vi "ADAM_kernal_server.vi"(0 "Board type":T2=enum."NB-MIO-16H", 1 "interval scanning":bool, 2 "Client Time":dbl, 5 "No of samples+extra":i32=128 min=0 step=1, 7 "Trigger mode":T1, 9 "output polarity":u16(ring)=1 items=["do not change", "positive", "negative"], 11 "Ch & spans":T3[](array[typedef]) {"low limit (-10V)" format="%.3f"; "high limit (10V)" format="%.3f"}, 12 "Actual Sampling rate (Hz)":dbl=1000.0 format="%.2f", 13 "Local Client?":bool, 14 "Current Block No":i32) -> (4 "I16 data":i16[][](array[numeric]), 6 "Block Timings":T4={"Started"=0.0, "Ended"=0.0, "Analogue Frequency Hz"=1000.0} {"Analogue Frequency Hz" format="%.2f"}, 10 "group channel settings":T5(array[cluster]) {"scale offset" format="%.2f"; "scale multiplier" format="%.2f"; "gain" format="%.2f"; "range" format="%.2f"; "lower input limits" format="%.2f"; "upper input limits" format="%.2f"}, 15 "error out":errorcluster)   [LabVIEW 2010]
uses:
  ADAM_Global.vi
  Anemometry/Anemometry Sub Vis/Globals/Meas_global.vi
  Anemometry/Anemometry Sub Vis/Controls/Block_start_and_end.ctl
  Channel_Description_Global.vi
  Anemometry/Anemometry Sub Vis/Globals/Constants_global.vi
  Anemometry/Anemometry Sub Vis/Controls/Board_Types.ctl
  Anemometry/Anemometry Sub Vis/Controls/Ch_and_Spans.ctl
  Anemometry/Anemometry Sub Vis/Controls/Trigger_Mode.ctl
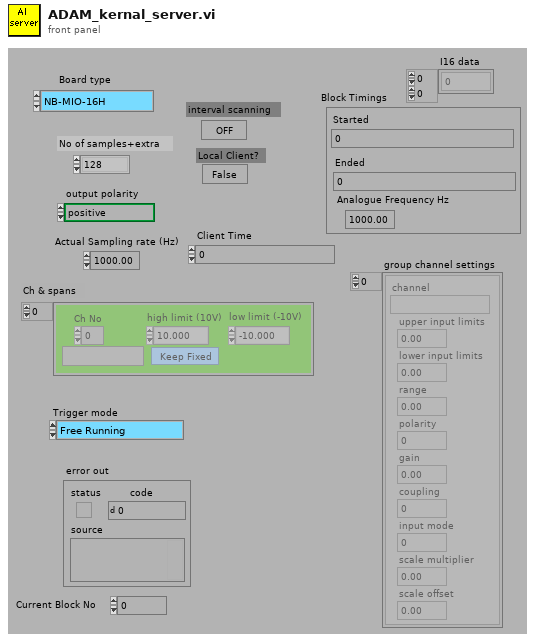
[diagram p1: front panel]
types:
  T1 = typedef "Trigger_Mode.ctl" = enum16{"Free Running", "Start on Trigger", "Trigger Every Block", "Trigger Every Sample"}
  T2 = typedef "Board_Types.ctl" = enum16{"Simulate", "NB-MIO-16H", "PCI-MIO-16E", "6000E Series", "USB-92xx", "ADC488", "Lab-NB", "NB-DIO-24", "NI-DAQmx", "Local ADAM", "Server Channels"}
  T3 = typedef "Ch_and_Spans.ctl" = cluster{"high limit (10V)":sgl, "low limit (-10V)":sgl, "Ch No":i16, "Var name":string, "Use Latest Calib":bool}
  T4 = typedef "Block_start_and_end.ctl" = cluster{"Started":dbl, "Ended":dbl, "Analogue Frequency Hz":dbl}
  T5 = cluster{"channel":string, "upper input limits":sgl, "lower input limits":sgl, "range":sgl, "polarity":u16, "gain":sgl, "coupling":u16, "input mode":u16, "scale multiplier":dbl, "scale offset":dbl}[]
  T6 = cluster{"channel":string, "upper input limits":sgl, "lower input limits":sgl, "range":sgl, "polarity":u16, "gain":sgl, "coupling":u16, "input mode":u16, "scale multiplier":dbl, "scale offset":dbl}
  T7 = typedef "Ch_description_ADAM.ctl" = cluster{"Ch Name":string, "Type":T8, "Function":T9, "Ch State":T10, "Calibration type":T11, "A":dbl, "B":dbl, "C":dbl, "D":dbl, "Comments":string, "Address":T12, "String":string, "Duty":u16}
  T8 = typedef "Module_type_ADAM.ctl" = enum16{"4011", "4012", "4013", "4014", "4016", "4017", "4018", "4021", "4050", "4052", "4053", "4060", "4080", "5000", "5017", "5018", "5024", "5051", "5056", "5060", "6060", "Tracker", "WEST", "GILL", "JEM", "VICI", "Vaisala", "DRUCK", "Run VI Named:", "IR2100", "PPT", "Comparator", "VIRTUAL", "Hold Value", "Read A", "Read Ch", "Coded", "Client Info", "Web Client", "X10", "Test"}
  T9 = typedef "Function_ADAM.ctl" = enum16{"Analogue Input", "Digital Input", "Event counter", "Event rate", "Analogue Output", "Digital Output", "Relay Output"}
  T10 = typedef "Channel_State.ctl" = enum16{"On", "Off", "Always On", "Always Off"}
  T11 = typedef "Calib_type_ADAM.ctl" = enum16{"Raw", "Bx + A", "Cx^2 + Bx + A", "Dx^3 + Cx^2 + Bx + A", "In Band", "Hi-Tec Q", "Hi-Tec M_dot", "Text"}
  T12 = typedef "Address.ctl" = cluster{"Main":i32, "Ch.":i32, "Sub":i32, "Port Name":string}
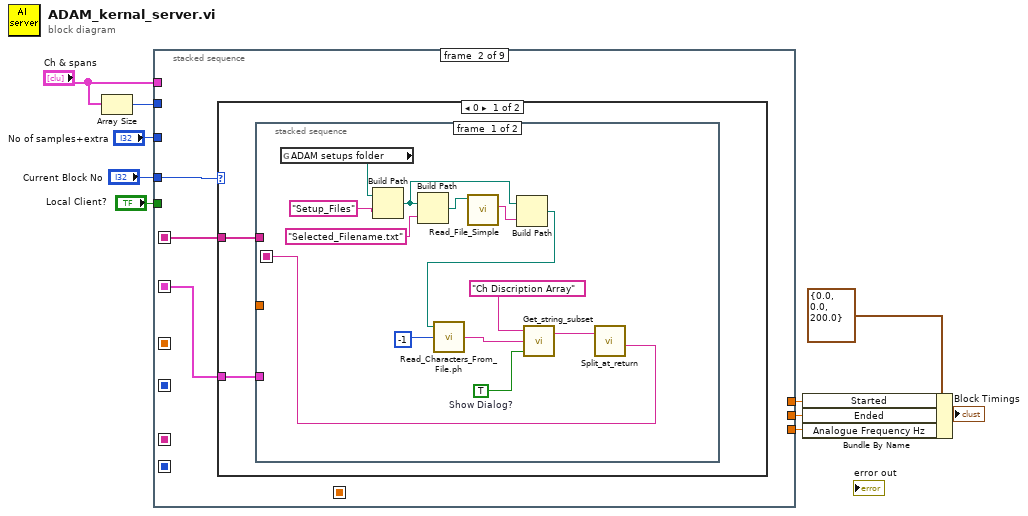
[diagram p0: block diagram]
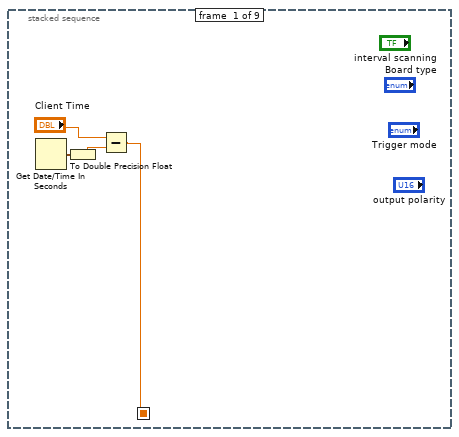
[diagram p2: hidden frame]
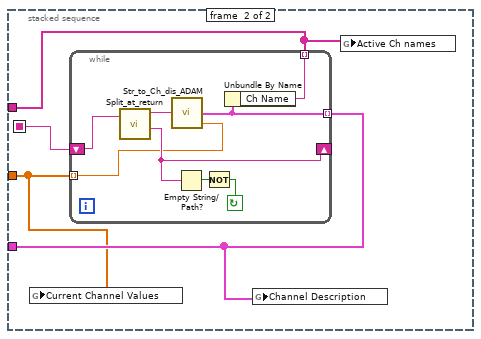
[diagram p3: hidden frame]
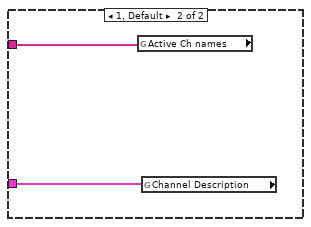
[diagram p4: hidden frame]
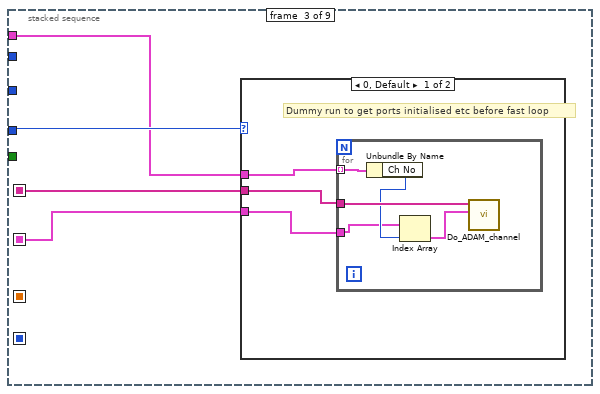
[diagram p5: hidden frame]
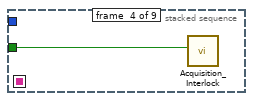
[diagram p7: hidden frame]
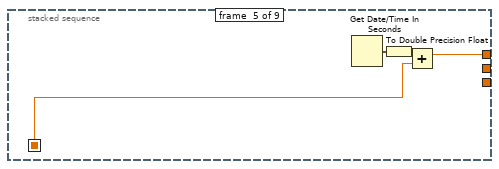
[diagram p8: hidden frame]
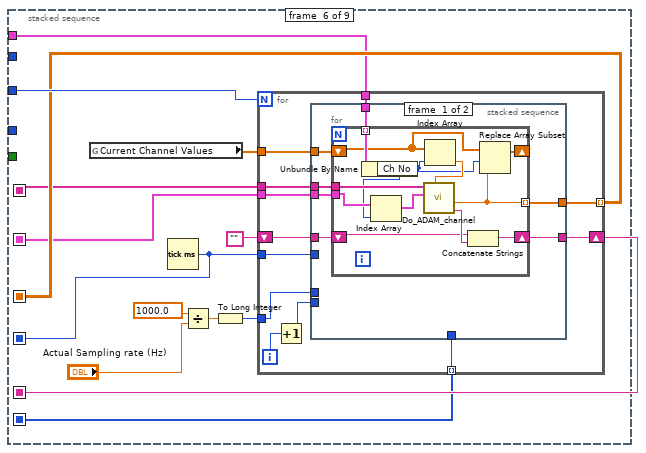
[diagram p9: hidden frame]
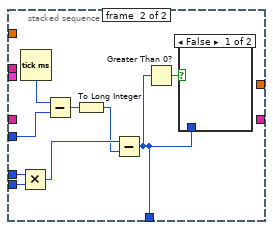
[diagram p10: hidden frame]
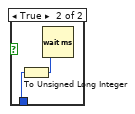
[diagram p11: hidden frame]
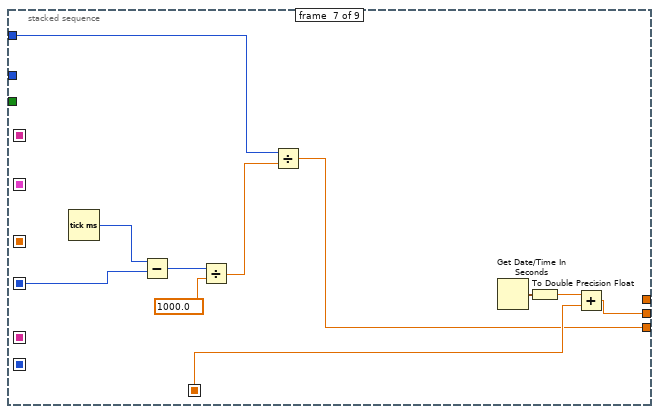
[diagram p12: hidden frame]
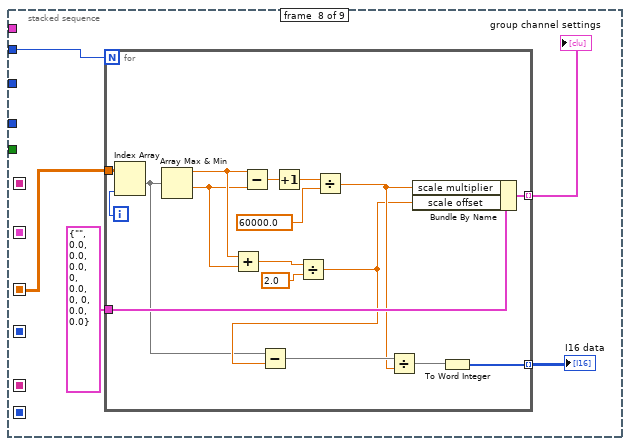
[diagram p13: hidden frame]
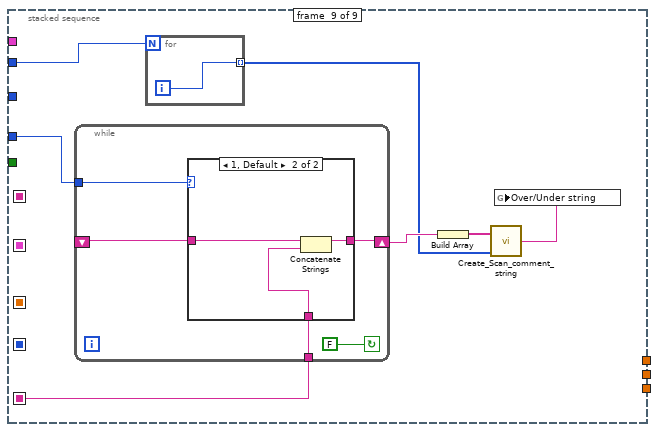
[diagram p14: hidden frame]
diagram:
  n1 = Array Size(array="Ch & spans") -> (size(s)=w2:i32)
  n2 = stacked-sequence {
    seq-local: [_ _ _ _ _ w75 _ _ _] -> [_ _ _ _ _ _ _ _ w159]
    seq-local: [_ _ _ _ _ w73 _ _ _] -> [_ _ _ _ _ _ _ w131 _]
    seq-local: [_ w16 _ _ _ _ _ _ _] -> [_ _ w50 _ _ w71 _ _ _]
    seq-local: [_ w17 _ _ _ _ _ _ _] -> [_ _ w49 _ _ w72 _ _ _]
    seq-local: [_ _ _ _ _ w70 _ _ _] -> [_ _ _ _ _ _ w130 _ _]
    seq-local: [_ _ _ _ _ w67 _ _ _] -> [_ _ _ _ _ _ _ _ _]
    seq-local: [w13 _ _ _ _ _ _ _ _] -> [_ _ _ _ w62 _ w123 _ _]
    tunnel: "No of samples+extra" -> [_ _ _ _ _ w74 w127 _ _]
    tunnel: "Current Block No" -> [_ w15 w48 _ _ _ _ _ w154]
    tunnel: [_ _ _ _ w61 _ _ _ _] -> w7
    tunnel: [_ _ _ _ _ _ w122 _ _] -> w6
    tunnel: "Local Client?" -> [_ _ _ w59 _ _ _ _ _]
    tunnel: "Ch & spans" -> [_ _ w47 _ _ w65 _ _ _]
    tunnel: w2 -> [_ _ _ _ _ _ _ w132 w153]
    tunnel: [_ _ _ _ _ _ w121 _ _] -> w1
    frame #0 {
      n3 = Get Date/Time In Seconds() -> (seconds since 1Jan1904=w11:timestamp)
      n4 = To Double Precision Float(number=w11) -> (double precision float=w14:dbl)
      n5 = Subtract(x="Client Time", y=w14) -> (x-y=w13:dbl)
    }
    frame #1 {
      n6 = case shown="0" w15 {
        tunnel: [w19 w46] -> w17
        tunnel: [w18 w45] -> w16
        frame 0 {
          n7 = stacked-sequence {
            seq-local: [w28 _] -> [_ w36]
            tunnel: [_ w35] -> w19
            tunnel: [_ w34] -> w18
            tunnel: [_ w33] -> _
            frame #0 {
              w27 = TRUE  # Show Dialog?
              n8 = global read "Constants_global.vi" "ADAM setups folder"() -> (w24:path)
              n9 = Build Path(base path=w24, name or relative path="Setup_Files") -> (appended path=w21:path)
              n10 = Build Path(base path=w21, name or relative path="Selected_Filename.txt" ("Substring")) -> (appended path=w23:path)
              n11 = call "Read_File_Simple.vi"("Filename"=w23) -> ("string"=w22:string)  [unwired: 4 in, 5 out]
              n12 = Build Path(base path=w21, name or relative path=w22) -> (appended path=w20:path)
              n13 = call "Read_Characters_From_File.ph.vi"("file path (dialog if empty)"=w20, "number of characters (all:-1)"=-1) -> ("character string"=w31:string)  [unwired: 4 in, 3 out]
              n14 = call "Get_string_subset.vi"("Show Dialog?"=w27, "String to split"=w31, "File Label"="Ch Discription Array") -> ("Output string"=w32:string)  [unwired: 1 out]
              n15 = call "Split_at_return.vi"("String"=w32) -> ("after substring"=w28:string)  [unwired: 1 in, 3 out]
            }
            frame #1 {
              n16 = while {
                tunnel: [w38] -> w35 mode=indexing
                tunnel: [w39] -> w34 mode=indexing
                shift-left: w36 -> [w44]
                shift-right: [w42] -> _
                tunnel: [w37] -> w33 mode=indexing
                stop <- w40 continue-if-true
                n17 = call "Split_at_return.vi"("String"=w44) -> ("before substring"=w43:string, "after substring"=w42:string)  [unwired: 1 in, 2 out]
                n18 = call "Str_to_Ch_dis_ADAM.vi"("String Row"=w43) -> ("Value"=w37:dbl, "Ch Description"=w39:T7)  [unwired: 3 in]
                n19 = Empty String/Path?(string/path=w42) -> (empty?=w41:bool)
                n20 = Not(x=w41) -> (.not. x?=w40:bool)
                n21 = Unbundle By Name(w39) -> ("Ch Name"=w38:string)
              }
              n22 = global write "ADAM_Global.vi" "Current Channel Values"(w33) -> ()
              n23 = global write "Channel_Description_Global.vi" "Channel Description"(w34) -> ()
              n24 = global write "ADAM_Global.vi" "Active Ch names"(w35) -> ()
            }
          }
        }
        frame 1, Default {
          n25 = global read "ADAM_Global.vi" "Active Ch names"() -> (w46:string[])
          n26 = global read "Channel_Description_Global.vi" "Channel Description"() -> (w45:T7[])
        }
      }
    }
    frame #2 {
      n27 = case shown="0, Default" w48 {
        tunnel: w50 -> [w53 _]
        tunnel: w49 -> [w52 _]
        tunnel: w47 -> [w51 _]
        frame 0, Default {
          # "Dummy run to get ports initialised etc before fast loop"
          n28 = for {
            tunnel: w53 -> [w54]
            tunnel: w52 -> [w57]
            tunnel: w51 -> [w58] mode=indexing
            n29 = Unbundle By Name(w58) -> ("Ch No"=w55:i16)
            n30 = Index Array(array=w54, index=w55) -> (element=w56:T7)
            n31 = call "Do_ADAM_channel.vi"("Ch Description"=w56, "Ch names"=w57) -> ()  [unwired: 6 in, 2 out]
          }
        }
        frame 1 {
        }
      }
    }
    frame #3 {
      n32 = call "Acquisition_Interlock.vi"("Local Control"=w59) -> ()
    }
    frame #4 {
      n33 = Get Date/Time In Seconds() -> (seconds since 1Jan1904=w60:timestamp)
      n34 = To Double Precision Float(number=w60) -> (double precision float=w63:dbl)
      n35 = Add(x=w63, y=w62) -> (x+y=w61:dbl)
    }
    frame #5 {
      n36 = global read "ADAM_Global.vi" "Current Channel Values"() -> (w64:dbl[])
      n37 = Tick Count (ms)() -> (millisecond timer value=w70:u32)
      n38 = Divide(x=1000.0 ("y"), y="Actual Sampling rate (Hz)") -> (x/y=w69:dbl)
      n39 = To Long Integer(number=w69) -> (32bit integer=w68:i32)
      n40 = for {
        N: w74 -> [_]
        tunnel: w71 -> [w89]
        tunnel: w72 -> [w88]
        tunnel: w68 -> [w82]
        shift-right: [w86] -> w75
        shift-left: "" -> [w87]
        tunnel: [w85] -> w73 mode=indexing
        tunnel: w70 -> [w84]
        tunnel: [w81] -> w67 mode=indexing
        tunnel: w65 -> [w79]
        tunnel: w64 -> [w78]
        i -> [w83]
        n41 = Increment(x=w83) -> (x+1=w80:i32)
        n42 = stacked-sequence {
          tunnel: w89 -> [w96 _]
          tunnel: w88 -> [w95 _]
          tunnel: w87 -> [w94 _]
          tunnel: [w93 _] -> w86
          tunnel: [w92 _] -> w85
          tunnel: w84 -> [_ w111]
          tunnel: w80 -> [_ w117]
          tunnel: w82 -> [_ w116]
          tunnel: [_ w115] -> w81
          tunnel: w79 -> [w91 _]
          tunnel: w78 -> [w90 _]
          frame #0 {
            n43 = for {
              tunnel: w96 -> [w103]
              tunnel: w95 -> [w108]
              shift-right: [w105] -> w93
              shift-left: w94 -> [w106]
              tunnel: [w98] -> w92 mode=indexing
              tunnel: w91 -> [w104] mode=indexing
              shift-right: [w97] -> _
              shift-left: w90 -> [w99]
              n44 = Unbundle By Name(w104) -> ("Ch No"=w100:i16)
              n45 = Index Array(array=w103, index=w100) -> (element=w102:T7)
              n46 = Index Array(array=w99, index=w100) -> (element=w101:dbl)
              n47 = call "Do_ADAM_channel.vi"("Previous Scan Value"=w101, "Ch Description"=w102, "Ch names"=w108) -> ("Scan comment"=w107:string, "Output"=w98:dbl)  [unwired: 5 in]
              n48 = Concatenate Strings(w106, w107) -> (w105:string)
              n49 = Replace Array Subset(array=w99, new element=w98, index=w100) -> (w97:dbl[])
            }
          }
          frame #1 {
            n50 = Multiply(x=w116, y=w117) -> (x*y=w110:i32)
            n51 = Tick Count (ms)() -> (millisecond timer value=w113:u32)
            n52 = Subtract(x=w113, y=w111) -> (x-y=w112:u32)
            n53 = To Long Integer(number=w112) -> (32bit integer=w109:i32)
            n54 = Subtract(x=w110, y=w109) -> (x-y=w115:i32)
            n55 = Greater Than 0?(x=w115) -> (x > 0?=w114:bool)
            n56 = case shown="False" w114 {
              tunnel: w115 -> [_ w119]
              frame False {
              }
              frame True {
                n57 = To Unsigned Long Integer(number=w119) -> (unsigned 32bit integer=w118:u32)
                n58 = Wait (ms)(milliseconds to wait=w118) -> ()  [unwired: 1 out]
              }
            }
          }
        }
      }
    }
    frame #6 {
      n59 = Tick Count (ms)() -> (millisecond timer value=w125:u32)
      n60 = Subtract(x=w125, y=w130) -> (x-y=w129:u32)
      n61 = Divide(x=w129, y=1000.0) -> (x/y=w126:dbl)
      n62 = Divide(x=w127, y=w126) -> (x/y=w121:dbl)
      n63 = Get Date/Time In Seconds() -> (seconds since 1Jan1904=w120:timestamp)
      n64 = To Double Precision Float(number=w120) -> (double precision float=w124:dbl)
      n65 = Add(x=w124, y=w123) -> (x+y=w122:dbl)
    }
    frame #7 {
      n66 = for {
        N: w132 -> [_]
        tunnel: T6 {"channel"="", "upper input limits"=0.0, "lower input limits"=0.0, "range"=0.0, "polarity"=0, "gain"=0.0, "coupling"=0, "input mode"=0, "scale multiplier"=0.0, "scale offset"=0.0} -> [w152]
        tunnel: [w151] -> w133 mode=indexing
        tunnel: [w144] -> w134 mode=indexing
        tunnel: w131 -> [w138]
        i -> [w137]
        n67 = Index Array(array=w138, index (col)=w137) -> (element=w136:dbl[])  [unwired: 1 in]
        n68 = Array Max & Min(array=w136) -> (max value=w149:dbl, min value=w148:dbl)  [unwired: 2 out]
        n69 = Add(x=w149, y=w148) -> (x+y=w147:dbl)
        n70 = Subtract(x=w149, y=w148) -> (x-y=w150:dbl)
        n71 = Increment(x=w150) -> (x+1=w142:dbl)
        n72 = Divide(x=w147, y=2.0) -> (x/y=w139:dbl)
        n73 = Subtract(x=w136, y=w139) -> (x-y=w141:dbl[])
        n74 = Divide(x=w142, y=60000.0) -> (x/y=w140:dbl)
        n75 = Divide(x=w141, y=w140) -> (x/y=w145:dbl[])
        n76 = Bundle By Name(cluster=w152, "scale multiplier"=w140, "scale offset"=w139) -> (w151:T6)
        n77 = To Word Integer(number=w145) -> (16bit integer=w144:i16[])
      }
      "I16 data" <- w134
      "group channel settings" <- w133
    }
    frame #8 {
      n78 = while {
        tunnel: w154 -> [w161]
        tunnel: w159 -> [w163]
        shift-left: _ -> [w162]
        shift-right: [w164] -> w157
        stop <- FALSE continue-if-true
        n79 = case shown="1, Default" w161 {
          tunnel: [w165 w166] -> w164
          tunnel: w163 -> [w165 w167]
          tunnel: w162 -> [_ w168]
          frame 0 {
          }
          frame 1, Default {
            n80 = Concatenate Strings(w168, w167) -> (w166:string)
          }
        }
      }
      n81 = for {
        N: w153 -> [_]
        tunnel: [w169] -> w156 mode=indexing
        i -> [w169]
      }
      n82 = Build Array(w157) -> (w158:string[])
      n83 = call "Create_Scan_comment_string.vi"("Requested channels"=w156, "Scan comments"=w158) -> ("Comment string"=w155:string)
      n84 = global write "Meas_global.vi" "Over/Under string"(w155) -> ()
    }
  }
  n85 = Bundle By Name(cluster=T4 {"Started"=0.0, "Ended"=0.0, "Analogue Frequency Hz"=200.0} ("Block Timings"), "Started"=w7, "Ended"=w6, "Analogue Frequency Hz"=w1) -> (→"Block Timings":T4)
